vi "LVClass_WavefrontCorrector Set Parameter Real.vi"(0 "WavefrontCorrector in":refnum<class "WavefrontCorrector.lvclass">, 5 "parameter_name":string, 9 "value":sgl, 11 "error in (no error)":errorcluster) -> (4 "WavefrontCorrector out":refnum<class "WavefrontCorrector.lvclass">, 15 "error out":errorcluster)   [LabVIEW 2020, in "WavefrontCorrector.lvclass"]
doc: "WavefrontCorrector parameter setter for parameter of type float.\n\n--------------------------------------------------------------------------------\n\n<B>correctorIn </B> : WavefrontCorrector object.\n<B>correctorOut </B> : WavefrontCorrector object.\n<B>parameter_name </B> : Name of the parameter.\n<B>value </B> : Value of the parameter.\n<B>ErrorIn </B> : Error\n<B>ErrorOut </B> : Error\n\n--------------------------------------------------------------------------------"
uses:
  WavefrontCorrector.lvclass
  WavefrontCorrector.lvclass/WavefrontCorrector.ctl
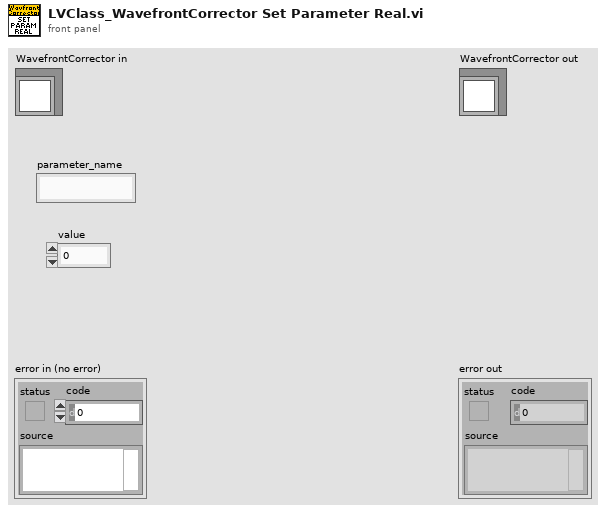
[diagram p1: front panel]
types:
  T1 = typedef "ClassID.ctl" = i64
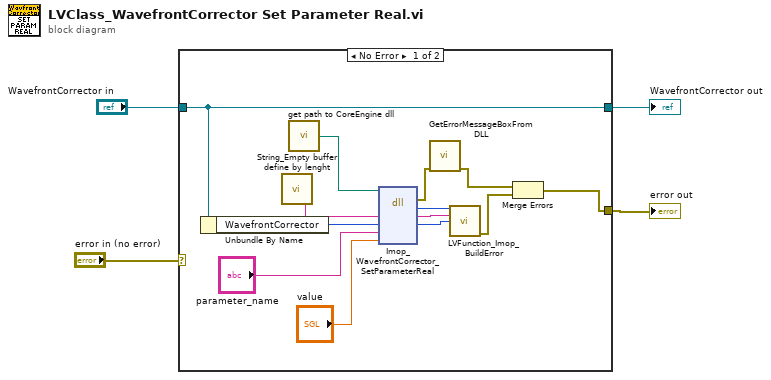
[diagram p0: block diagram]
diagram:
  n1 = case shown="No Error" "error in (no error)" {
    selector: "error in (no error)" -> [_ w19]
    tunnel: [w6 w19] -> w2
    tunnel: [w13 w18] -> w1
    tunnel: "WavefrontCorrector in" -> [w13 w18]
    frame No Error {
      n2 = Unbundle By Name(w13) -> ("WavefrontCorrector"=w14:T1)
      n3 = call "String_Empty buffer define by lenght.vi"() -> ("Empty buffer"=w17:string)  [unwired: 1 in]
      n4 = call "get path to CoreEngine dll.vi"() -> ("path to wavekit library"=w12:path)  [unwired: 14 in, 1 out]
      n5 = dll-call lib="D:/soft/HASO_v3/SVN_trunk/ImOpCoreEngine4_LV2011/DLLs/c_interface_vc100.dll" fn="Imop_WavefrontCorrector_SetParameterReal"(path in=w12, "message"=w17, "camera"=w14, "parameter_name"="parameter_name", "value"="value") -> (error out=w11:errorcluster, "return type"=w16:i32, "message"=w15:string, "camera"=w5:i64)  [unwired: 4 in, 1 out]
      n6 = call "GetErrorMessageBoxFromDLL.vi"("error IN"=w11) -> ("error OUT"=w8:errorcluster)  [unwired: 10 in]
      n7 = call "LVFunction_Imop_BuildError.vi"("code"=w16, "String to Prepend to source (\"\")"=w15, "Adresse"=w5) -> ("error out"=w7:errorcluster)  [unwired: 12 in]
      n8 = Merge Errors(w8, w7) -> (w6:errorcluster)
    }
    frame Error {
    }
  }
  "error out" <- w2
  "WavefrontCorrector out" <- w1
